vi "ID.vi"(11 "WT1600.lvlib:WT1600.lvclass":refnum<class "WT1600.lvclass">) -> (2 "Full ID":string, 3 "WT1600.lvlib:WT1600.lvclass 2":refnum<class "WT1600.lvclass">)   [LabVIEW 2013, in "WT1600.lvlib" / "WT1600.lvclass"]
uses:
  WT1600.lvclass
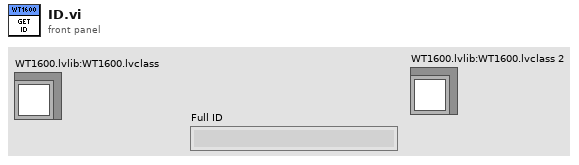
[diagram p1: front panel]
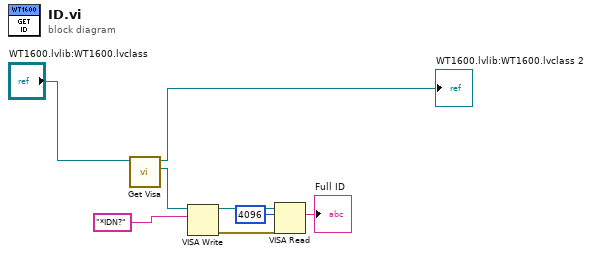
[diagram p0: block diagram]
diagram:
  n1 = call "Get Visa.vi"("WT1600.lvlib:WT1600.lvclass"="WT1600.lvlib:WT1600.lvclass") -> ("WT1600 Visa"=w4:refnum<visa-resource-name>, "WT1600.lvlib:WT1600.lvclass 2"=→"WT1600.lvlib:WT1600.lvclass 2":refnum<class "WT1600.lvclass">)  [unwired: 9 in]
  n2 = VISA Write(VISA resource name=w4, write buffer="*IDN?") -> (VISA resource name out=w8:refnum<visa-resource-name>, error out=w7:errorcluster)  [unwired: 1 in, 1 out]
  n3 = VISA Read(VISA resource name=w8, byte count=u32 4096, error in (no error)=w7) -> (read buffer=→"Full ID":string)  [unwired: 3 out]
